vi "SRV_Number of IMJ Requests Methods.vi"(0 "Number of IMJ Requests ref":refnum<vi>, 1 "semaphore ref":T1, 11 "error in (no error)":errorcluster, 12 "Number of IMJ Requests Methods (Read)":T2) -> (3 "semaphore ref out":T1, 4 "Number of IMJ Requests ref out":refnum<vi>, 8 "Number of IMJ Requests":i32, 10 "Zero Requests?":bool, 15 "error out":errorcluster)   [LabVIEW 2009]
doc: "Manages the value of a global \"Number of IMJ Requests\". A semaphore needs to be acquired to prevent race conditions in updating the number.\n\n\nAuthor: Mike Schultz - Logic PD"
uses:
  SRV_Number of IMJ Requests Methods.ctl
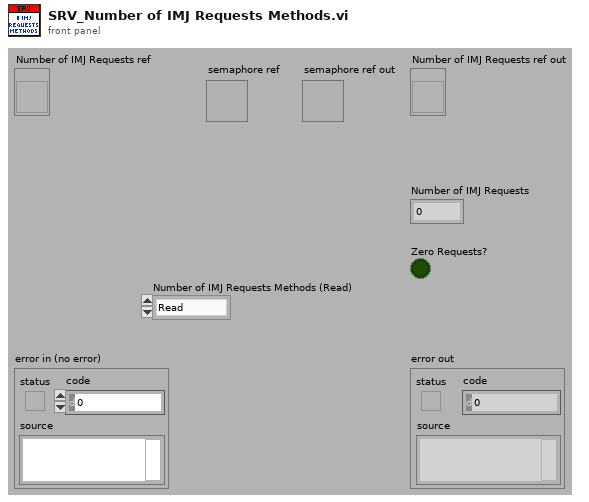
[diagram p1: front panel]
types:
  T1 = typedef "Semaphore RefNum" = refnum<k1>
  T2 = typedef "SRV_Number of IMJ Requests Methods.ctl" = enum16{"Read", "Increment", "Decrement", "Reset", "Close"}
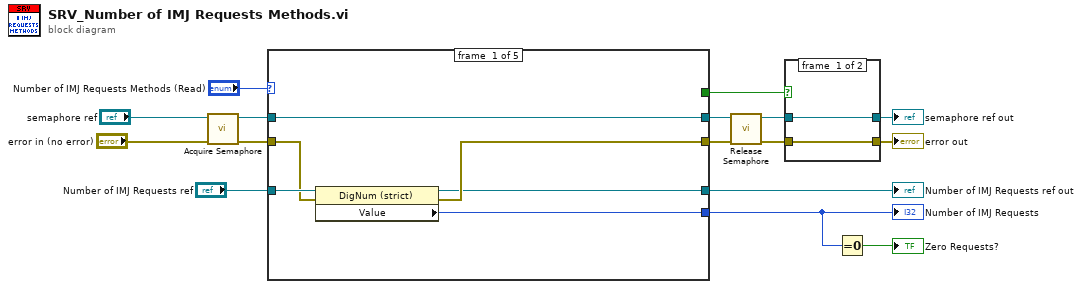
[diagram p0: block diagram]
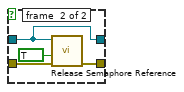
[diagram p2: hidden frame]
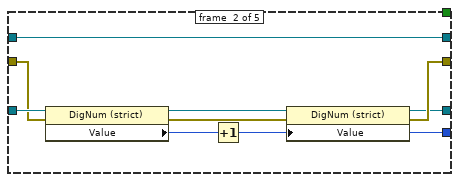
[diagram p3: hidden frame]
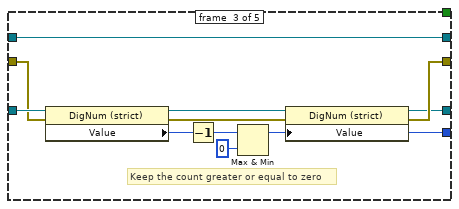
[diagram p4: hidden frame]
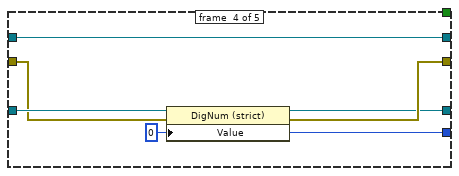
[diagram p5: hidden frame]
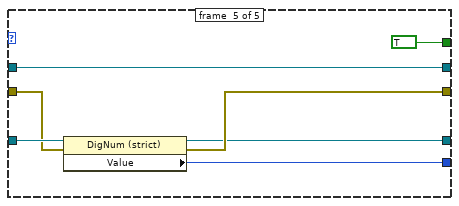
[diagram p6: hidden frame]
diagram:
  n1 = call <vilib>:"Acquire Semaphore.vi"("error in (no error)"="error in (no error)", "semaphore"="semaphore ref") -> ("error out"=w15:errorcluster, "semaphore out"=w16:T1)  [unwired: 3 in, 1 out]
  n2 = case shown="\"Decrement\"" "Number of IMJ Requests Methods (Read)" {
    tunnel: w16 -> [w22 w31 w42 w48 w55]
    tunnel: w15 -> [w20 w29 w40 w44 w52]
    tunnel: "Number of IMJ Requests ref" -> [w21 w30 w41 w45 w53]
    tunnel: [w22 w31 w42 w48 w55] -> w13
    tunnel: [w19 w25 w36 w47 w51] -> w12
    tunnel: [w18 w24 w35 w46 w50] -> w10
    tunnel: [_ _ _ _ TRUE] -> w2
    tunnel: [w17 w23 w32 w43 w49] -> w6
    frame #0 {
      n3 = property class="DigNum (strict)"(reference=w21, error in=w20) -> (reference out=w18:refnum<vi>, error out=w19:errorcluster, "Value"=w17:i32)
    }
    frame #1 {
      n4 = property class="DigNum (strict)"(reference=w30, error in=w29) -> (reference out=w28:refnum<vi>, error out=w27:errorcluster, "Value"=w26:i32)
      n5 = Increment(x=w26) -> (x+1=w23:i32)
      n6 = property class="DigNum (strict)"(reference=w28, error in=w27, "Value"=w23) -> (reference out=w24:refnum<vi>, error out=w25:errorcluster)
    }
    frame #2 {
      # "Keep the count greater or equal to zero"
      n7 = property class="DigNum (strict)"(reference=w41, error in=w40) -> (reference out=w39:refnum<vi>, error out=w38:errorcluster, "Value"=w37:i32)
      n8 = Decrement(x=w37) -> (x-1=w33:i32)
      n9 = Max & Min(x=w33, y=0) -> (max(x,y)=w32:i32)  [unwired: 1 out]
      n10 = property class="DigNum (strict)"(reference=w39, error in=w38, "Value"=w32) -> (reference out=w35:refnum<vi>, error out=w36:errorcluster)
    }
    frame #3 {
      w43 = 0 ("Value")
      n11 = property class="DigNum (strict)"(reference=w45, error in=w44, "Value"=w43) -> (reference out=w46:refnum<vi>, error out=w47:errorcluster)
    }
    frame #4 {
      n12 = property class="DigNum (strict)"(reference=w53, error in=w52) -> (reference out=w50:refnum<vi>, error out=w51:errorcluster, "Value"=w49:i32)
    }
  }
  "Number of IMJ Requests ref out" <- w10
  "Number of IMJ Requests" <- w6
  n13 = call <vilib>:"Release Semaphore.vi"("error in (no error)"=w12, "semaphore"=w13) -> ("error out"=w9:errorcluster, "semaphore out"=w7:T1)  [unwired: 4 in]
  n14 = case shown="True" w2 {
    tunnel: w9 -> [w57 w61]
    tunnel: [w57 w60] -> w8
    tunnel: w7 -> [w56 w58]
    tunnel: [w56 w58] -> w1
    frame #0 {
    }
    frame #1 {
      n15 = call <vilib>:"Release Semaphore Reference.vi"("error in (no error)"=w61, "force destroy? (F)"=TRUE, "semaphore"=w58) -> ("error out"=w60:errorcluster)  [unwired: 7 in, 1 out]
    }
  }
  "error out" <- w8
  "semaphore ref out" <- w1
  n16 = Equal To 0?(x=w6) -> (x = 0?=→"Zero Requests?":bool)
